vi "字符串清除回车换行.vi"(8 "error in (no error)":errorcluster, 11 "输入字符串":string) -> (0 "error out":errorcluster, 3 "输出字符串":string)   [LabVIEW 2020]
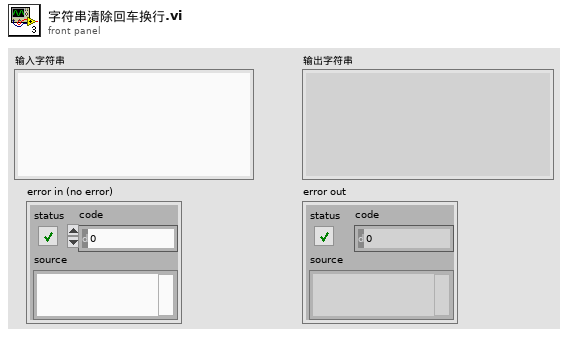
[diagram p1: front panel]
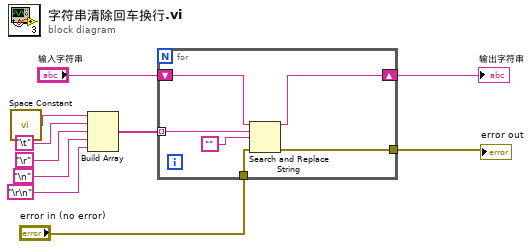
[diagram p0: block diagram]
diagram:
  n1 = call <vilib>:"Space Constant.vi"() -> ("String"=w10:string)
  n2 = Build Array(w10, "\t", "\r", "\n", "\r\n") -> (w5:string[])
  n3 = for {
    tunnel: w5 -> [w16] mode=indexing
    shift-right: [w13] -> w3
    shift-left: "输入字符串" -> [w14]
    tunnel: "error in (no error)" -> [w12]
    tunnel: [w11] -> w1
    n4 = Search and Replace String(input string=w14, search string=w16, replace string="", error in=w12) -> (result string=w13:string, error out=w11:errorcluster)  [unwired: 4 in, 2 out]
  }
  "输出字符串" <- w3
  "error out" <- w1
